vi "lab_3_pre_lab.vi"() -> ()   [LabVIEW 2016]
panel:
  out "raw data file":refnum<file>
  out "Folder_Name":string
  in  "DATE":string
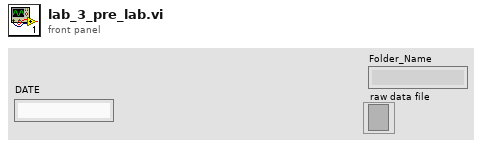
[diagram p1: front panel]
types:
  T1 = enum16{"open", "replace", "create", "open or create", "replace or create", "replace or create with confirmation"}
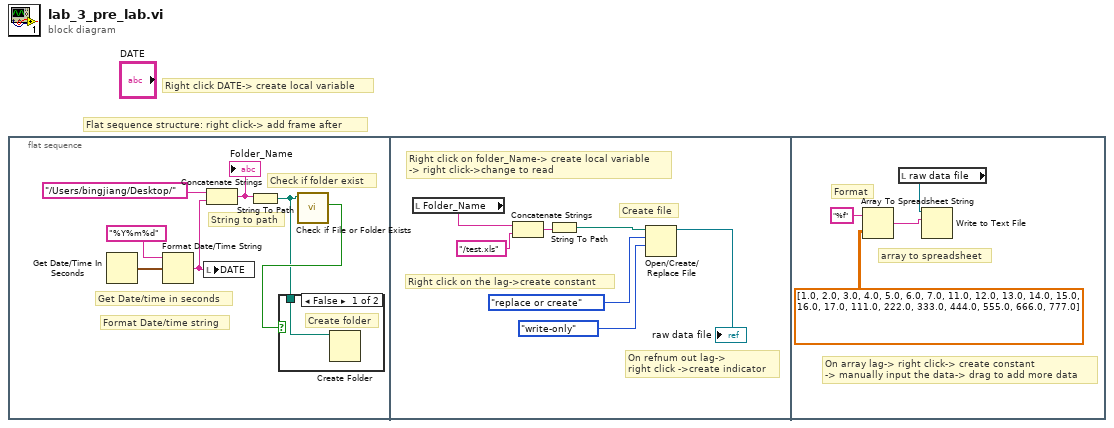
[diagram p0: block diagram]
diagram:
  # "Right click DATE-> create local variable"
  # "Flat sequence structure: right click-> add frame after"
  n1 = flat-sequence {
    frame #0 {
      # "Check if folder exist"
      # "String to path"
      # "Get Date/time in seconds"
      # "Format Date/time string"
      n2 = Get Date/Time In Seconds() -> (seconds since 1Jan1904=w7:timestamp)
      n3 = Format Date/Time String(time format string (%c)="%Y%m%d", seconds (now)=w7) -> (date/time string=w5:string)  [unwired: 1 in]
      n4 = local write "DATE"(w5) -> ()
      n5 = Concatenate Strings("/Users/bingjiang/Desktop/" ("string"), w5) -> (w3:string)
      "Folder_Name" <- w3
      n6 = String To Path(string=w3) -> (path=w1:path)
      n7 = call <vilib>:"Check if File or Folder Exists.vi"("path"=w1) -> ("file or folder exists?"=w2:bool)  [unwired: 8 in, 2 out]
      n8 = case shown="False" w2 {
        tunnel: w1 -> [w8 _]
        frame False {
          # "Create folder"
          n9 = Create Folder(path (use dialog)=w8) -> ()  [unwired: 2 in, 3 out]
        }
        frame True {
        }
      }
    }
    frame #1 {
      # "On refnum out lag->\nright click ->create indicator"
      # "Right click on the lag->create constant"
      # "Create file"
      # "Right click on folder_Name-> create local variable\n-> right click->change to read"
      n10 = local read "Folder_Name"() -> (w15:string)
      n11 = Concatenate Strings(w15, "/test.xls") -> (w13:string)
      n12 = String To Path(string=w13) -> (path=w12:path)
      n13 = Open/Create/Replace File(file path (use dialog)=w12, operation (0:open)=T1."replace or create", access (0:read/write)=enum16{"read/write", "read-only", "write-only"}."write-only") -> (refnum out=→"raw data file":refnum<file>)  [unwired: 3 in, 2 out]
    }
    frame #2 {
      # "On array lag-> right click-> create constant\n-> manually input the data-> drag to add more data"
      # "Format"
      # "array to spreadsheet"
      n14 = Array To Spreadsheet String(array=dbl[][] [[1.0, 2.0, 3.0, 4.0, 5.0, 6.0, 7.0], [11.0, 12.0, 13.0, 14.0, 15.0, 16.0, 17.0], [111.0, 222.0, 333.0, 444.0, 555.0, 666.0, 777.0]], 3:"%f" ("format string")) -> (spreadsheet string=w19:string)  [unwired: 1 in]
      n15 = local read "raw data file"() -> (w17:refnum<file>)
      n16 = Write to Text File(file (use dialog)=w17, text=w19) -> ()  [unwired: 2 in, 3 out]
    }
  }
